vi "ResetTable Result (SubVI).vi"(11 "Table in":refnum<vi>) -> ()   [LabVIEW 2017]
uses:
  <vilib>/Utility/miscctls.llb/LVRowAndColumnTypeDef.ctl
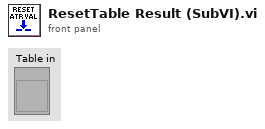
[diagram p1: front panel]
types:
  T1 = typedef "LVRowAndColumnTypeDef.ctl" = cluster{"Row":i32, "Column":i32}
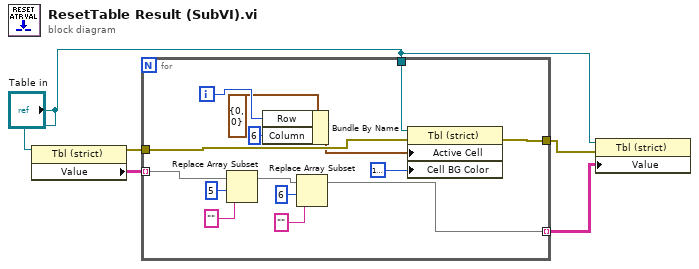
[diagram p0: block diagram]
diagram:
  n1 = property class="Tbl (strict)"(reference="Table in") -> (error out=w5:errorcluster, "Value"=w4:string[][])  [unwired: 1 in, 1 out]
  n2 = for {
    tunnel: w5 -> [w19]
    tunnel: [w18] -> w1
    tunnel: "Table in" -> [w17]
    tunnel: w4 -> [w12] mode=indexing
    tunnel: [w6] -> w3 mode=indexing
    i -> [w20]
    n3 = Replace Array Subset(array=w12, new element="" ("new element/subarray"), index=5) -> (w7:string[])
    n4 = Bundle By Name(cluster=T1 {"Row"=0, "Column"=0} ("Active Cell:Active Cell"), "Row"=w20, "Column"=6) -> (w14:T1)
    n5 = Replace Array Subset(array=w7, new element="" ("new element/subarray"), index=6) -> (w6:string[])
    n6 = property class="Tbl (strict)"(reference=w17, error in=w19, "Active Cell"=w14, "Cell BG Color"=u32 16777226) -> (error out=w18:errorcluster)  [unwired: 1 out]
  }
  n7 = property class="Tbl (strict)"(reference="Table in", error in=w1, "Value"=w3) -> ()  [unwired: 2 out]
